vi "Insert SP.vi"(8 "error in (no error)":errorcluster, 10 "VI Ref":refnum<vi>, 11 "Subpanel-Abstract in":refnum<class "Subpanel-Abstract.lvclass">) -> (0 "error out":errorcluster, 3 "Subpanel-Abstract out":refnum<class "Subpanel-Abstract.lvclass">)   [LabVIEW 2023, in "Data Analysis.lvlib" / "Subpanel-Abstract.lvclass"]
uses:
  Subpanel-Abstract.lvclass
  Subpanel-Abstract.lvclass/Subpanel-Abstract.ctl
  <vilib>/Utility/miscctls.llb/LVPointTypeDef.ctl
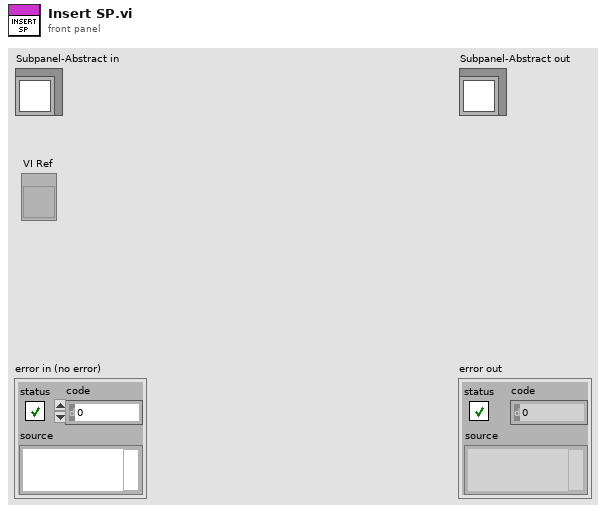
[diagram p1: front panel]
types:
  T1 = typedef "LVPointTypeDef.ctl" = cluster{"Horizontal":i16, "Vertical":i16}
  T2 = enum16{"Always On", "Always Off", "Off While Running"}
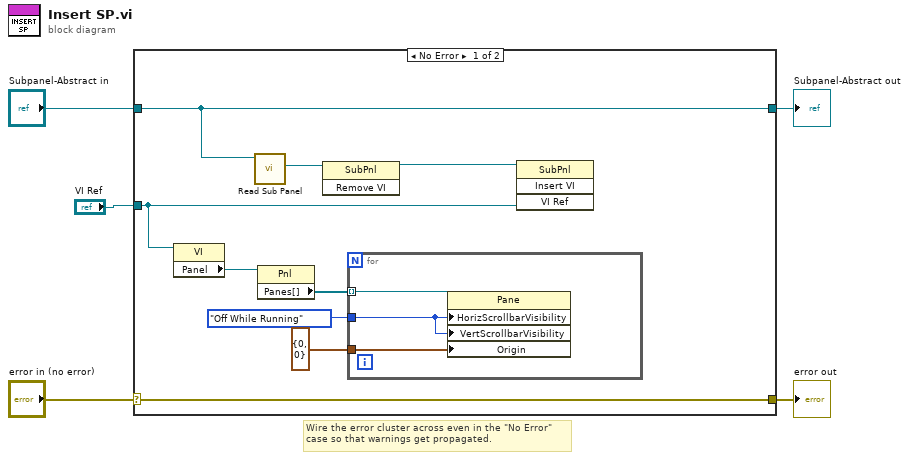
[diagram p0: block diagram]
diagram:
  # "Wire the error cluster across even in the \"No Error\"\ncase so that warnings get propagated."
  n1 = case shown="No Error" "error in (no error)" {
    selector: "error in (no error)" -> [w14 w19]
    tunnel: [w14 w19] -> w4
    tunnel: [w13 w18] -> w2
    tunnel: "Subpanel-Abstract in" -> [w13 w18]
    tunnel: "VI Ref" -> [w10 _]
    frame No Error {
      n2 = property class="VI"(reference=w10) -> ("Panel"=w9:refnum<vi>)  [unwired: 1 in, 2 out]
      n3 = call "Read Sub Panel.vi"("Subpanel-Abstract in"=w13) -> ("Sub Panel"=w12:refnum<vi>)  [unwired: 8 in, 2 out]
      n4 = property class="Pnl"(reference=w9) -> ("Panes[]"=w8:refnum<vi>[])  [unwired: 1 in, 2 out]
      n5 = invoke class="SubPnl" method="Remove VI"(reference=w12) -> (reference out=w11:refnum<vi>)  [unwired: 2 in, 2 out]
      n6 = for {
        tunnel: w8 -> [w17] mode=indexing
        tunnel: T2."Off While Running" ("Horizontal Scrollbar Visibility") -> [w16]
        tunnel: T1 {"Horizontal"=0, "Vertical"=0} ("Origin") -> [w15]
        n7 = property class="Pane"(reference=w17, "HorizScrollbarVisibility"=w16, "VertScrollbarVisibility"=w16, "Origin"=w15) -> ()  [unwired: 1 in, 2 out]
      }
      n8 = invoke class="SubPnl" method="Insert VI"(reference=w11, "VI Ref"=w10) -> ()  [unwired: 2 in, 4 out]
    }
    frame Error {
    }
  }
  "error out" <- w4
  "Subpanel-Abstract out" <- w2
